vi "Mean_fr_NaN_data.vi"(0 "Data":dbl[](array[numeric]) format="%.2f") -> (1 "Mean value":dbl format="%.2f", 2 "GoodFraction":dbl)   [LabVIEW 2012]
uses:
  <vilib>/Analysis/baseanly.llb/Mean (DBL).vi
  <vilib>/Analysis/NI_AALBase.lvlib
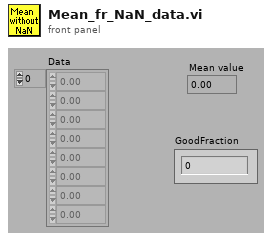
[diagram p1: front panel]
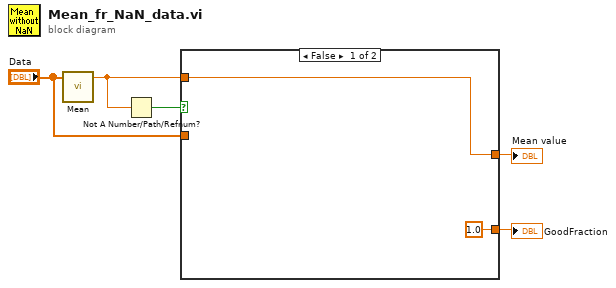
[diagram p0: block diagram]
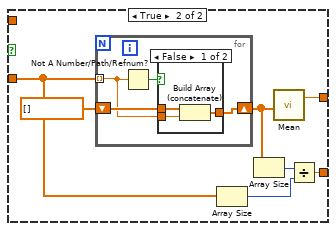
[diagram p2: hidden frame]
diagram:
  n1 = call-poly <vilib>:"Mean.vi"("X"="Data") -> ("mean"=w3:dbl)  [unwired: 1 out]
  n2 = Not A Number/Path/Refnum?(number/path/refnum=w3) -> (NaN/Path/Refnum?=w2:bool)
  n3 = case shown="False" w2 {
    tunnel: "Data" -> [_ w11]
    tunnel: [w7 w14] -> w4
    tunnel: w3 -> [w7 _]
    tunnel: [1.0 w8] -> w1
    frame False {
    }
    frame True {
      n4 = for {
        tunnel: w11 -> [w15] mode=indexing
        shift-right: [w17] -> w12
        shift-left: dbl[] [] -> [w18]
        n5 = Not A Number/Path/Refnum?(number/path/refnum=w15) -> (NaN/Path/Refnum?=w16:bool)
        n6 = case shown="False" w16 {
          tunnel: w18 -> [w21 w22]
          tunnel: [w20 w22] -> w17
          tunnel: w15 -> [w19 _]
          frame False {
            n7 = Build Array (concatenate)(w21, w19) -> (w20:dbl[])
          }
          frame True {
          }
        }
      }
      n8 = Array Size(array=w11) -> (size(s)=w9:i32)
      n9 = Array Size(array=w12) -> (size(s)=w10:i32)
      n10 = call-poly <vilib>:"Mean.vi"("X"=w12) -> ("mean"=w14:dbl)  [unwired: 1 out]
      n11 = Divide(x=w10, y=w9) -> (x/y=w8:dbl)
    }
  }
  "Mean value" <- w4
  "GoodFraction" <- w1
